vi "CalcCMR.vi"(8 "Zero?":bool, 10 "Load Sensors":dbl[](array[numeric]), 11 "Ref Sensor":dbl) -> (3 "delta SNS":dbl)   [LabVIEW 2013]
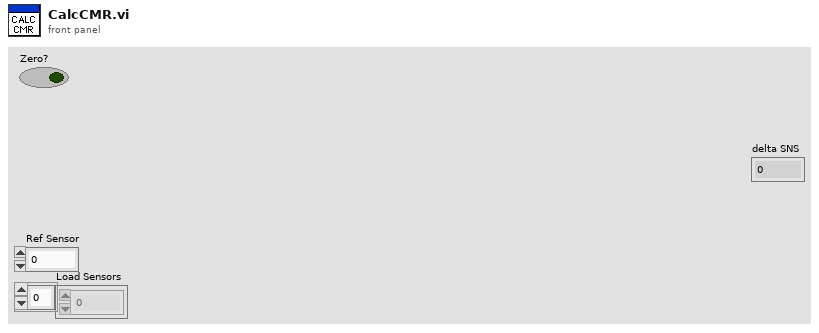
[diagram p1: front panel]
types:
  T1 = cluster{"SNS":dbl, "delta SNS":dbl, "zero SNS":dbl}
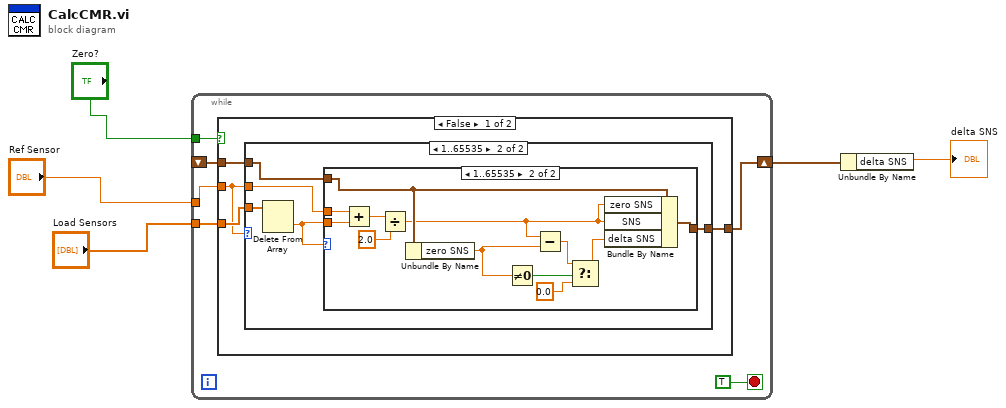
[diagram p0: block diagram]
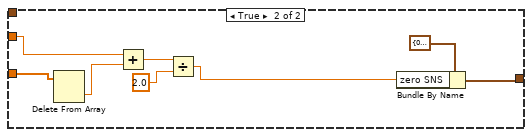
[diagram p4: hidden frame]
diagram:
  n1 = while {
    tunnel: "Load Sensors" -> [w10]
    tunnel: "Ref Sensor" -> [w9]
    tunnel: "Zero?" -> [w8]
    shift-right: [w11] -> w4
    shift-left: _ -> [w7]
    stop <- TRUE stop-if-true
    n2 = case shown="False" w8 {
      tunnel: [w15 w42] -> w11
      tunnel: w7 -> [w14 _]
      tunnel: w10 -> [w13 w38]
      tunnel: w9 -> [w12 w41]
      frame False {
        n3 = case shown="1..65535" w12 {
          tunnel: w12 -> [_ w21]
          tunnel: w13 -> [_ w20]
          tunnel: [w16 w19] -> w15
          tunnel: w14 -> [w16 w17]
          frame 0, Default {
          }
          frame 1..65535 {
            n4 = Delete From Array(array=w20) -> (deleted portion=w18:dbl)  [unwired: 2 in, 1 out]
            n5 = case shown="1..65535" w18 {
              tunnel: w18 -> [_ w33]
              tunnel: w21 -> [_ w31]
              tunnel: [w22 w30] -> w19
              tunnel: w17 -> [w22 w29]
              frame 0, Default {
              }
              frame 1..65535 {
                n6 = Add(x=w31, y=w33) -> (x+y=w34:dbl)
                n7 = Divide(x=w34, y=2.0) -> (x/y=w28:dbl)
                n8 = Unbundle By Name(w29) -> ("zero SNS"=w27:dbl)
                n9 = Not Equal To 0?(x=w27) -> (x != 0?=w26:bool)
                n10 = Subtract(x=w28, y=w27) -> (x-y=w25:dbl)
                n11 = Select(t=w25, s=w26, f=0.0) -> (s? t:f=w24:dbl)
                n12 = Bundle By Name(cluster=w29, "zero SNS"=w28, "SNS"=w28, "delta SNS"=w24) -> (w30:T1)
              }
            }
          }
        }
      }
      frame True {
        n13 = Delete From Array(array=w38) -> (deleted portion=w37:dbl)  [unwired: 2 in, 1 out]
        n14 = Add(x=w41, y=w37) -> (x+y=w40:dbl)
        n15 = Divide(x=w40, y=2.0) -> (x/y=w36:dbl)
        n16 = Bundle By Name(cluster=T1 {"SNS"=0.0, "delta SNS"=0.0, "zero SNS"=0.0} ("SNS"), "zero SNS"=w36) -> (w42:T1)
      }
    }
  }
  n17 = Unbundle By Name(w4) -> ("delta SNS"=→"delta SNS":dbl)
